vi "General Config.vi"(8 "error In":errorcluster, 10 "IOList":T2, 11 "reference":refnum<vi>) -> (0 "error out":errorcluster, 3 "Out reference":refnum<vi>)   [LabVIEW 2015]
uses:
  Control Button/Exit.ctl
  Control Button/Daq.ctl
  Control Button/Scanner config.ctl
  Control Button/Program Seq.ctl
  Control Button/cali.ctl
  Control Button/shift change.ctl
  Control Button/User mgt.ctl
  Control Button/model create.ctl
  Galobal variable_TI.vi
panel:
  in  "lvdt Setting":bool
  out "Job Id":string
  in  "image Setting":bool
  out "User Name 3":string
  in  "Model Create":T1
  in  "User Mgt":T3
  out "User Name 2":string
  in  "Shift":T4
  in  "Calibration":T5
  in  "IO List Update":bool
  out "error out 2":errorcluster
  in  "error in (no error)":errorcluster
  in  "Program Seq":T6
  in  "Scanner config":T7
  in  "DAQ Config":T8
  out "User Name":string
  in  "Exit":T9
  out "String":string
  out "appended path":path
  in  "Ring":u16(ring)
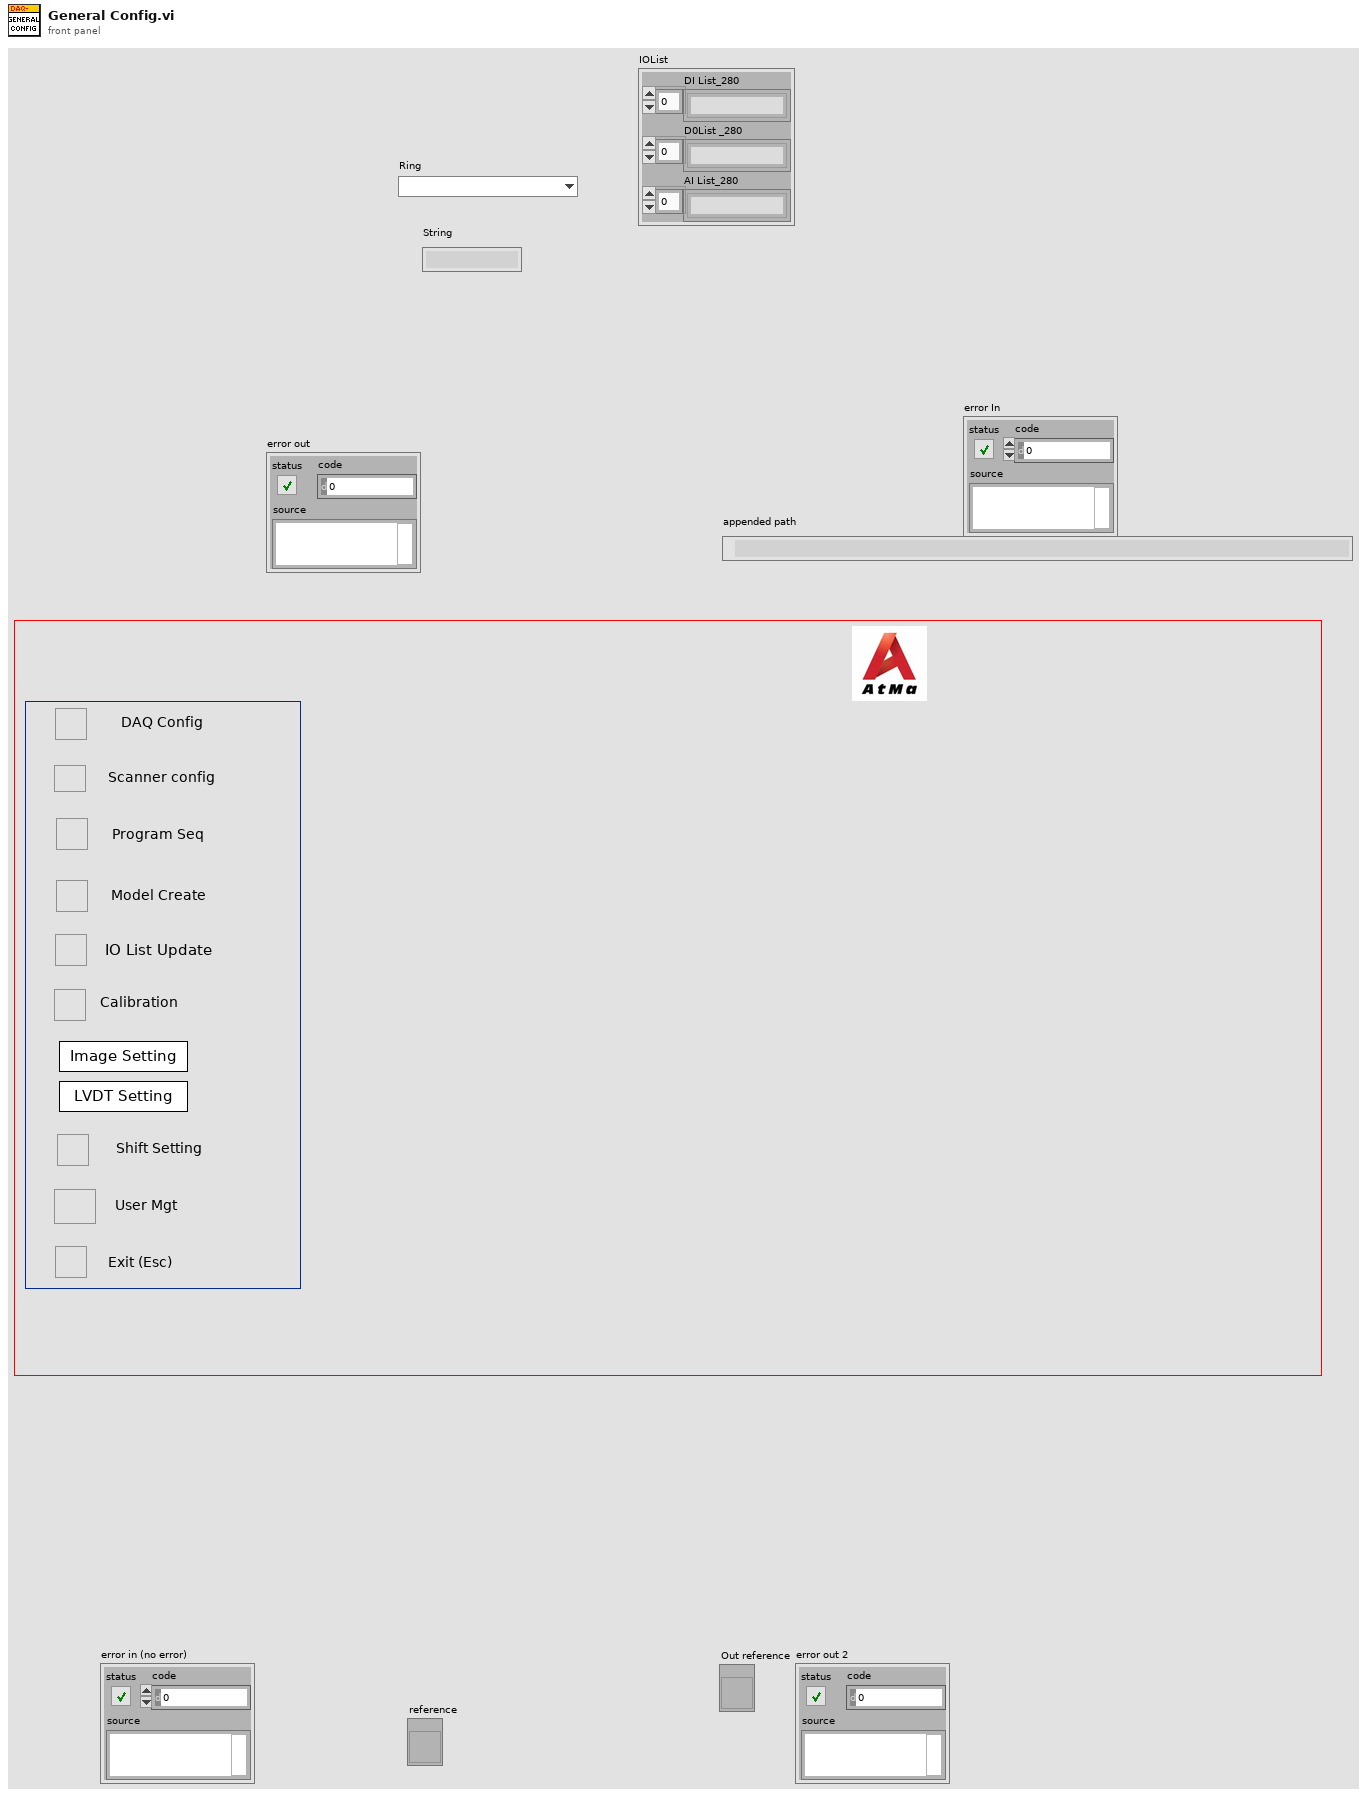
[diagram p1: front panel]
types:
  T1 = typedef "model create.ctl" = bool
  T2 = cluster{"DI List_280":string[], "D0List _280":string[], "AI List_280":string[]}
  T3 = typedef "User mgt.ctl" = bool
  T4 = typedef "shift change.ctl" = bool
  T5 = typedef "cali.ctl" = bool
  T6 = typedef "Program Seq.ctl" = bool
  T7 = typedef "Scanner config.ctl" = bool
  T8 = typedef "Daq.ctl" = bool
  T9 = typedef "Exit.ctl" = bool
  T10 = enum32{"Invalid", "Standard", "Closed", "Hidden", "Minimized", "Maximized"}
  T11 = cluster{"XInput":dbl[], "Y New Value":dbl[], "Avg point":i16}[]
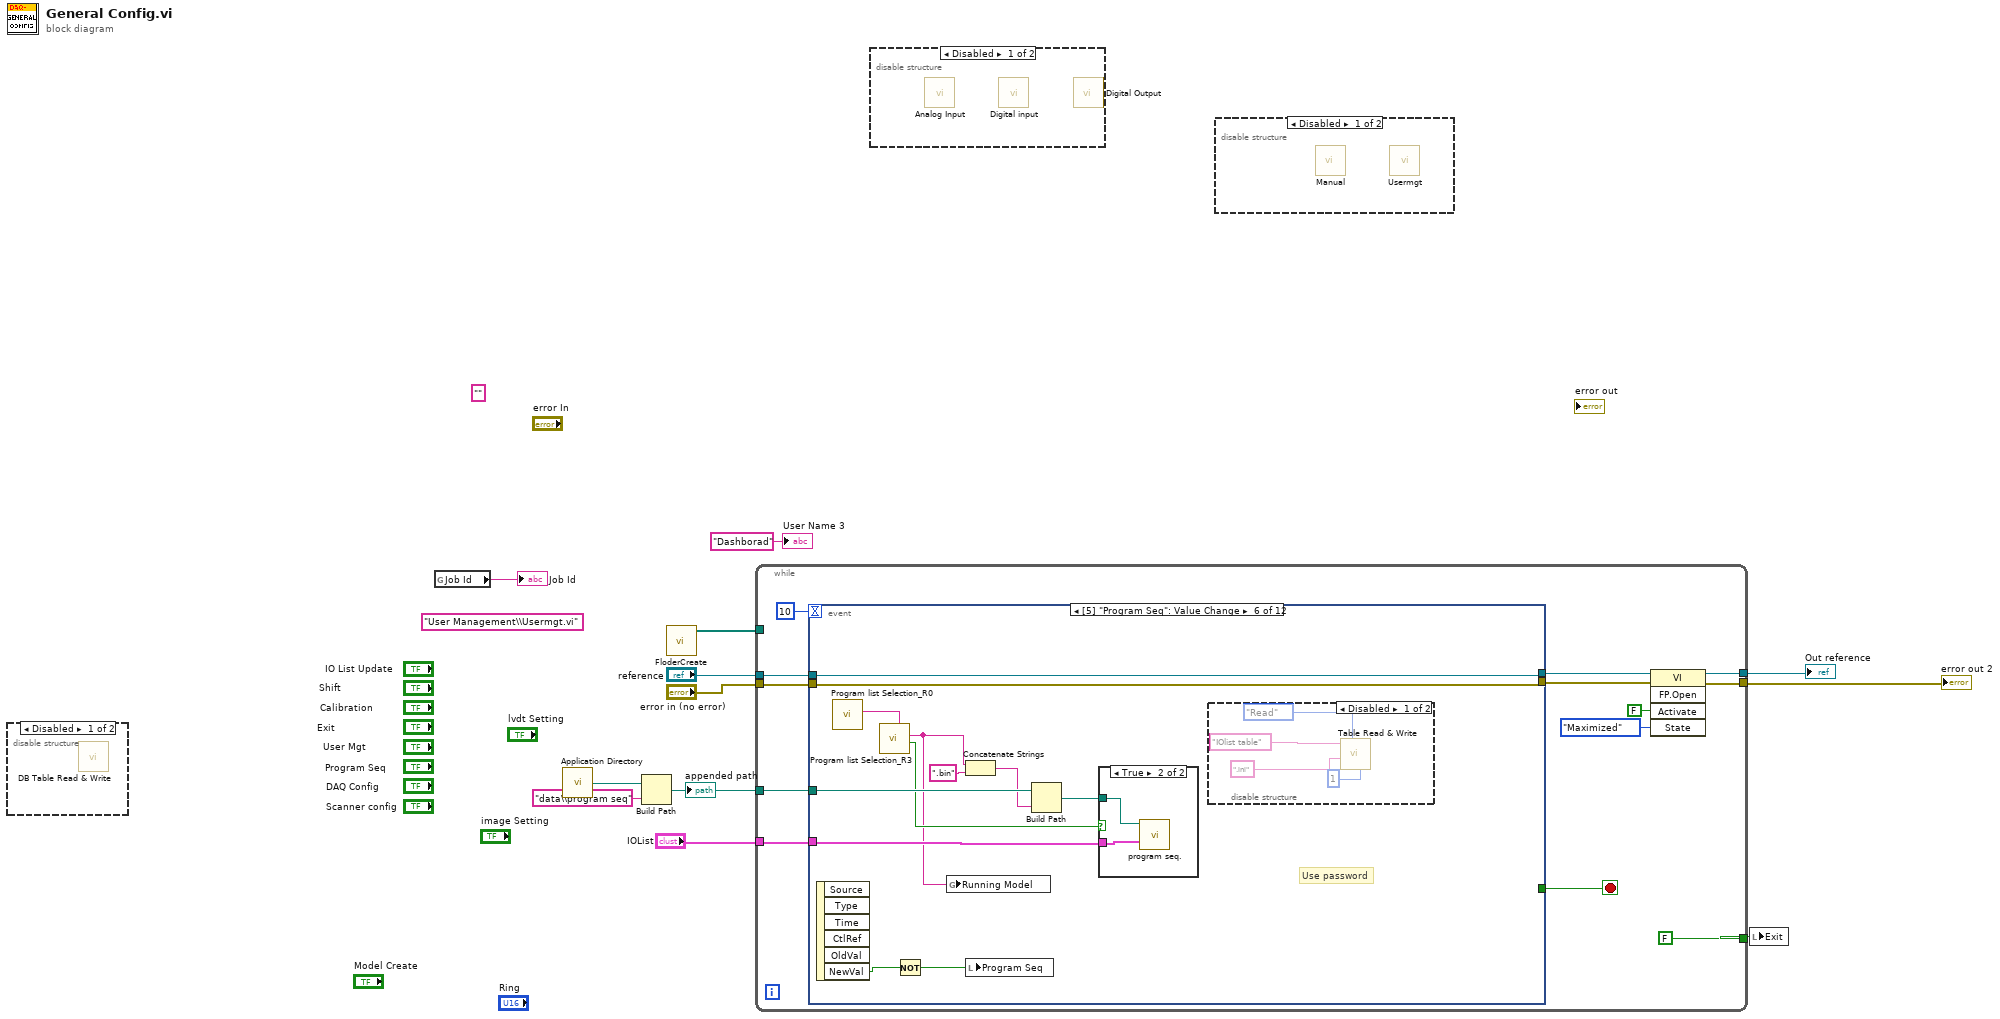
[diagram p0: block diagram]
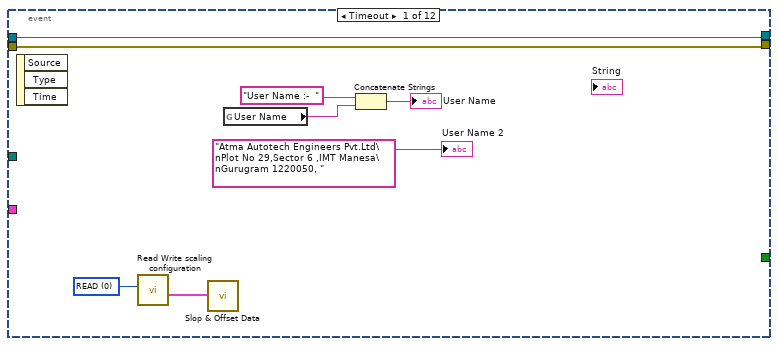
[diagram p5: hidden frame]
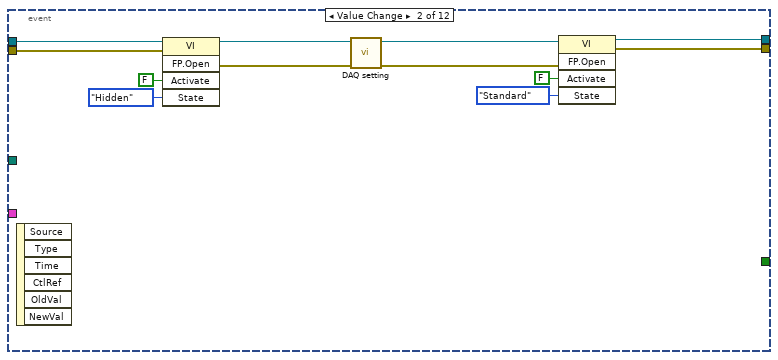
[diagram p6: hidden frame]
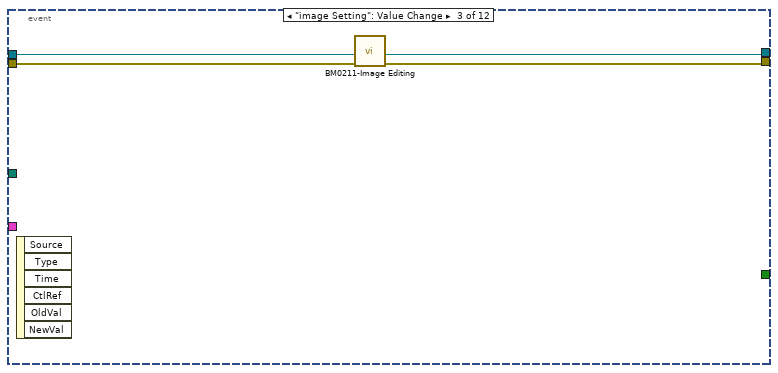
[diagram p7: hidden frame]
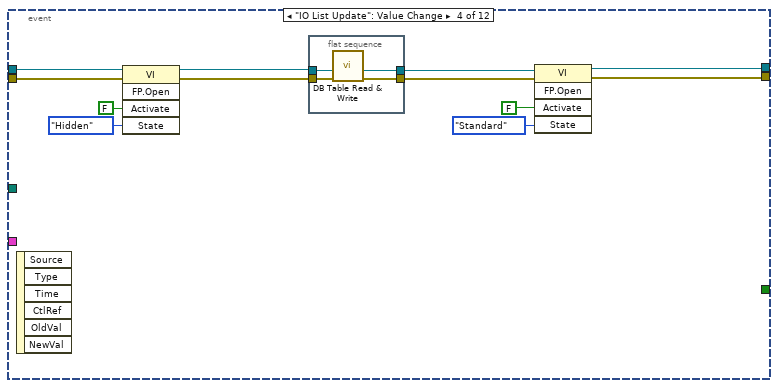
[diagram p8: hidden frame]
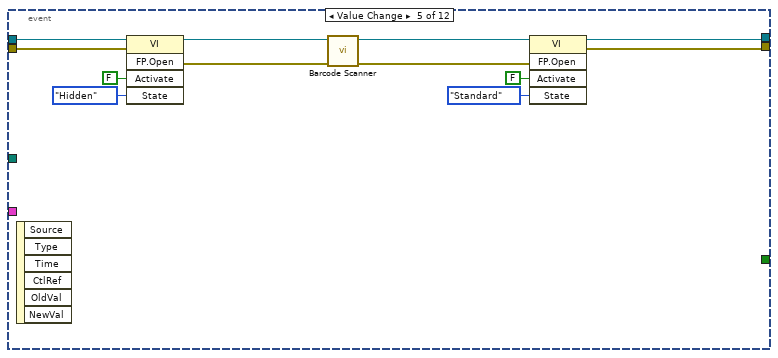
[diagram p9: hidden frame]
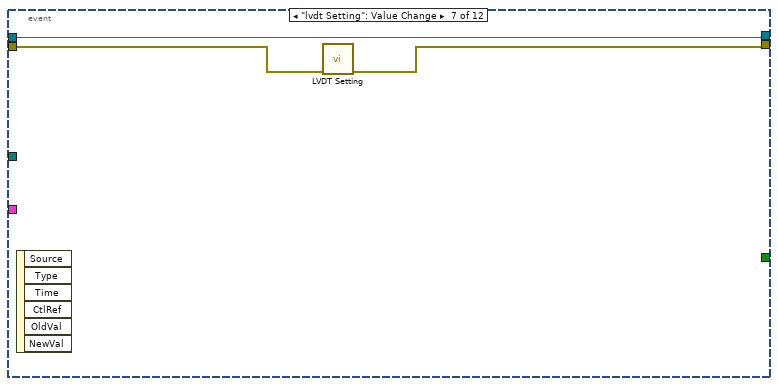
[diagram p12: hidden frame]
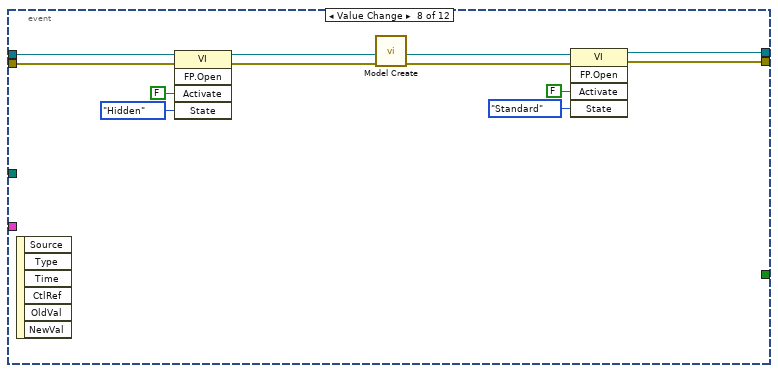
[diagram p13: hidden frame]
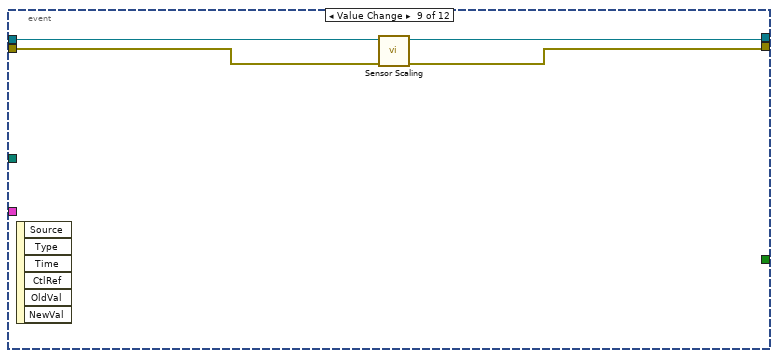
[diagram p14: hidden frame]
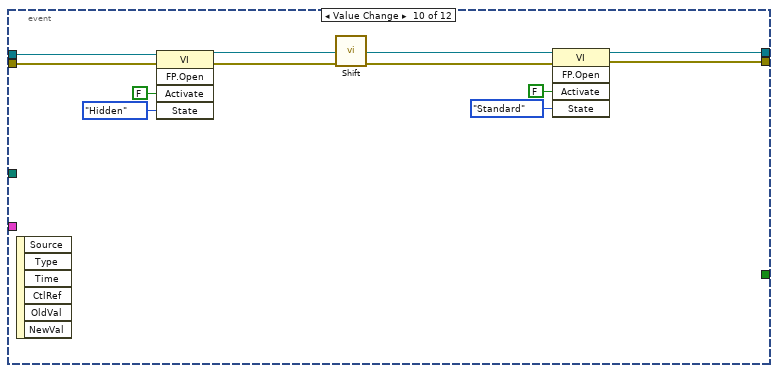
[diagram p15: hidden frame]
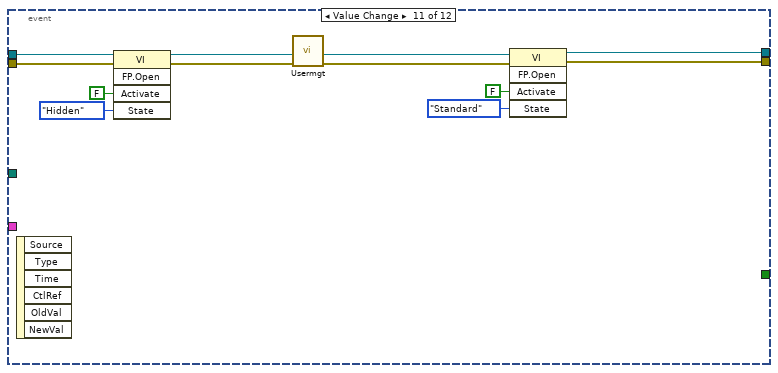
[diagram p16: hidden frame]
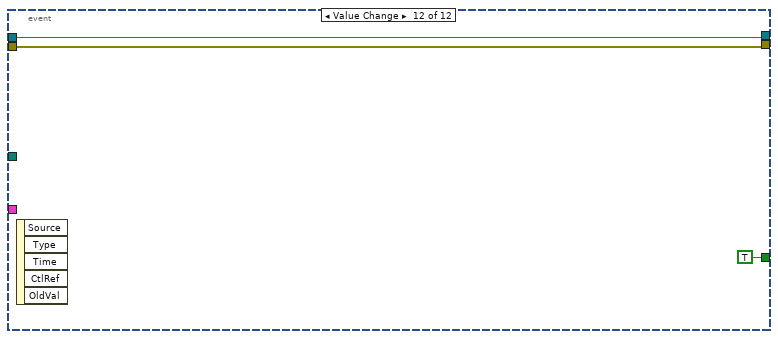
[diagram p17: hidden frame]
diagram:
  (unwired) "User Management\\Usermgt.vi" ("name or relative path")
  (unwired) ""
  n1 = disable-structure shown="Disabled" {
    frame Disabled {
      n2 = call "DB Table Read & Write.vi"() -> ()  [unwired: 10 in, 2 out]
    }
    frame Enabled {
    }
  }
  n3 = global read "Galobal variable_TI.vi" "Job Id"() -> (→"Job Id":string)
  n4 = call <vilib>:"Application Directory.vi"() -> ("Application Directory"=w6:path)
  n5 = Build Path(base path=w6, name or relative path="data\\program seq") -> (appended path=w3:path)
  "appended path" <- w3
  n6 = call "FloderCreate.vi"() -> ("File Path"=w7:path[])  [unwired: 11 in]
  n7 = while {
    tunnel: w3 -> [w13]
    tunnel: "reference" -> [w23]
    tunnel: "error in (no error)" -> [w22]
    tunnel: [w17] -> w11
    tunnel: [w16] -> w10
    tunnel: [T9 FALSE ("Exit")] -> w9
    tunnel: w7 -> [_]
    tunnel: "IOList" -> [w14]
    stop <- w24 stop-if-true
    n8 = event shown="[5] \"Program Seq\": Value Change" {
      selector: _ -> [_ _ _ _ _ _ _ _ _ _ _ _]
      dyn-events: _ -> [_ _ _ _ _ _ _ _ _ _ _ _]
      timeout: 10 -> [_ _ _ _ _ _ _ _ _ _ _ _]
      tunnel: [_ _ _ _ _ _ _ _ _ _ _ TRUE ("Exit")] -> w24
      tunnel: w23 -> [w30 w37 w48 w52 w74 w88 w97 w104 w111 w119 w128 w136]
      tunnel: w22 -> [w29 w36 w47 w51 w73 w87 w96 w103 w110 w117 w126 w135]
      tunnel: [w30 w35 w48 w59 w66 w88 w97 w99 w111 w118 w127 w136] -> w19
      tunnel: [w29 w34 w46 w58 w65 w87 w95 w98 w109 w116 w125 w135] -> w18
      tunnel: w14 -> [_ _ _ _ _ w86 _ _ _ _ _ _]
      tunnel: w13 -> [_ _ _ _ _ w85 _ _ _ _ _ _]
      event Timeout {
        w28 = u16 0 items=["READ", "WRITE"] ("Read/Write")
        n9 = event-data() -> ()  [unwired: 1 in, 3 out]
        n10 = call "Read Write scaling configuration.vi"("Read/Write"=w28) -> ("Output"=w27:T11)  [unwired: 4 in, 2 out]
        n11 = call "Slop & Offset Data.vi"("Input"=w27) -> ()  [unwired: 10 in, 1 out]
        n12 = global read "Galobal variable_TI.vi" "User Name"() -> (w33:string)
        n13 = Concatenate Strings("User Name :-  " ("string"), w33) -> (→"User Name":string)
        "User Name 2" <- "Atma Autotech Engineers Pvt.Ltd\nPlot No 29,Sector 6 ,IMT Manesa\nGurugram 1220050, " ("string")
      }
      event Value Change {
        n14 = event-data() -> ()  [unwired: 1 in, 6 out]
        n15 = invoke class="VI" method="FP.Open"(reference=w37, error in=w36, "Activate"=FALSE ("Activate?"), "State"=T10."Hidden") -> (reference out=w43:refnum<vi>, error out=w42:errorcluster)  [unwired: 1 in, 3 out]
        n16 = call "DAQ setting.vi"("error in (no error)"=w42, "vi reference"=w43) -> ("error Out"=w38:errorcluster, "Out reference"=w39:refnum<vi>)  [unwired: 8 in]
        n17 = invoke class="VI" method="FP.Open"(reference=w39, error in=w38, "Activate"=FALSE ("Activate?"), "State"=T10."Standard") -> (reference out=w35:refnum<vi>, error out=w34:errorcluster)  [unwired: 1 in, 3 out]
      }
      event "image Setting": Value Change {
        n18 = event-data() -> ()  [unwired: 1 in, 6 out]
        n19 = call "BM0211-Image Editing.vi"("error IN"=w47) -> ("error out"=w46:errorcluster)  [unwired: 10 in]
      }
      event "IO List Update": Value Change {
        n20 = event-data() -> ()  [unwired: 1 in, 6 out]
        n21 = invoke class="VI" method="FP.Open"(reference=w52, error in=w51, "Activate"=FALSE ("Activate?"), "State"=T10."Hidden") -> (reference out=w50:refnum<vi>, error out=w49:errorcluster)  [unwired: 1 in, 3 out]
        n22 = flat-sequence {
          tunnel: [w61] -> w56
          tunnel: [w62] -> w55
          tunnel: w50 -> [w63]
          tunnel: w49 -> [w64]
          frame #0 {
            n23 = call "DB Table Read & Write.vi"("error in"=w64, "reference"=w63) -> ("error out"=w61:errorcluster, "referenceOut"=w62:refnum<vi>)  [unwired: 8 in]
          }
        }
        n24 = invoke class="VI" method="FP.Open"(reference=w55, error in=w56, "Activate"=FALSE ("Activate?"), "State"=T10."Standard") -> (reference out=w59:refnum<vi>, error out=w58:errorcluster)  [unwired: 1 in, 3 out]
      }
      event Value Change {
        n25 = event-data() -> ()  [unwired: 1 in, 6 out]
        n26 = invoke class="VI" method="FP.Open"(reference=w74, error in=w73, "Activate"=FALSE ("Activate?"), "State"=T10."Hidden") -> (reference out=w70:refnum<vi>, error out=w69:errorcluster)  [unwired: 1 in, 3 out]
        n27 = call "Barcode Scanner.vi"("error in (no error)"=w69, "reference"=w70) -> ("error in (no error) 2"=w67:errorcluster, "reference 2"=w68:refnum<vi>)  [unwired: 8 in]
        n28 = invoke class="VI" method="FP.Open"(reference=w68, error in=w67, "Activate"=FALSE ("Activate?"), "State"=T10."Standard") -> (reference out=w66:refnum<vi>, error out=w65:errorcluster)  [unwired: 1 in, 3 out]
      }
      event Value Change {
        # "Use password"
        n29 = event-data() -> ("NewVal"=w81:T6)  [unwired: 1 in, 5 out]
        n30 = call "Program list Selection_R0.vi"() -> ("String"=w79:string)  [unwired: 8 in, 3 out]
        n31 = call "Program list Selection_R3.vi"("new element/subarray"=w79) -> ("Exit"=w78:bool, "String"=w77:string)  [unwired: 7 in, 2 out]
        n32 = Not(x=w81) -> (.not. x?=w80:T6)
        n33 = global write "Galobal variable_TI.vi" "Running Model"(w77) -> ()
        n34 = Concatenate Strings(w77, ".bin" ("string")) -> (w84:string)
        n35 = local write "Program Seq"(w80) -> ()
        n36 = Build Path(base path=w85, name or relative path=w84) -> (appended path=w82:path)
        n37 = case shown="True" w78 {
          tunnel: w86 -> [_ w89]
          tunnel: w82 -> [_ w90]
          frame False {
          }
          frame True {
            n38 = call "program seq..vi"("IOList"=w89, "Filepath"=w90) -> ()  [unwired: 9 in, 1 out]
          }
        }
        n39 = disable-structure shown="Disabled" {
          frame Disabled {
            n40 = call "Table Read & Write.vi"("File Name"="IOlist table", "File type"=".ini", "Enum"=enum16{"Read", "Write"}."Read", "index"=1) -> ()  [unwired: 5 in, 2 out]
          }
          frame Enabled {
          }
        }
      }
      event "lvdt Setting": Value Change {
        n41 = event-data() -> ()  [unwired: 1 in, 6 out]
        n42 = call "LVDT Setting.vi"("error in (no error)"=w96) -> ("error out 2"=w95:errorcluster)  [unwired: 10 in]
      }
      event Value Change {
        n43 = event-data() -> ()  [unwired: 1 in, 6 out]
        n44 = invoke class="VI" method="FP.Open"(reference=w104, error in=w103, "Activate"=FALSE ("Activate?"), "State"=T10."Hidden") -> (reference out=w100:refnum<vi>, error out=w102:errorcluster)  [unwired: 1 in, 3 out]
        n45 = call "Model Create.vi"("error in (no error)"=w102) -> ("error out"=w101:errorcluster)  [unwired: 10 in]
        n46 = invoke class="VI" method="FP.Open"(reference=w100, error in=w101, "Activate"=FALSE ("Activate?"), "State"=T10."Standard") -> (reference out=w99:refnum<vi>, error out=w98:errorcluster)  [unwired: 1 in, 3 out]
      }
      event Value Change {
        n47 = event-data() -> ()  [unwired: 1 in, 6 out]
        n48 = call "Sensor Scaling.vi"("error in"=w110) -> ("error out"=w109:errorcluster)  [unwired: 9 in, 1 out]
      }
      event Value Change {
        n49 = event-data() -> ()  [unwired: 1 in, 6 out]
        n50 = invoke class="VI" method="FP.Open"(reference=w119, error in=w117, "Activate"=FALSE ("Activate?"), "State"=T10."Hidden") -> (reference out=w120:refnum<vi>, error out=w122:errorcluster)  [unwired: 1 in, 3 out]
        n51 = call "Shift.vi"("error in"=w122) -> ("error out"=w121:errorcluster)  [unwired: 10 in]
        n52 = invoke class="VI" method="FP.Open"(reference=w120, error in=w121, "Activate"=FALSE ("Activate?"), "State"=T10."Standard") -> (reference out=w118:refnum<vi>, error out=w116:errorcluster)  [unwired: 1 in, 3 out]
      }
      event Value Change {
        n53 = event-data() -> ()  [unwired: 1 in, 6 out]
        n54 = invoke class="VI" method="FP.Open"(reference=w128, error in=w126, "Activate"=FALSE ("Activate?"), "State"=T10."Hidden") -> (reference out=w129:refnum<vi>, error out=w124:errorcluster)  [unwired: 1 in, 3 out]
        n55 = call "Usermgt.vi"("error In"=w124) -> ("error out"=w123:errorcluster)  [unwired: 10 in]
        n56 = invoke class="VI" method="FP.Open"(reference=w129, error in=w123, "Activate"=FALSE ("Activate?"), "State"=T10."Standard") -> (reference out=w127:refnum<vi>, error out=w125:errorcluster)  [unwired: 1 in, 3 out]
      }
      event Value Change {
        n57 = event-data() -> ()  [unwired: 1 in, 5 out]
      }
    }
    n58 = invoke class="VI" method="FP.Open"(reference=w19, error in=w18, "Activate"=FALSE ("Activate?"), "State"=T10."Maximized") -> (reference out=w17:refnum<vi>, error out=w16:errorcluster)  [unwired: 1 in, 3 out]
  }
  "Out reference" <- w11
  "error out 2" <- w10
  n59 = disable-structure shown="Disabled" {
    frame Disabled {
      n60 = call "Analog Input.vi"() -> ()  [unwired: 10 in, 2 out]
      n61 = call "Digital input.vi"() -> ()  [unwired: 10 in, 2 out]
      n62 = call "Digital Output.vi"() -> ()  [unwired: 10 in, 2 out]
    }
    frame Enabled {
    }
  }
  n63 = disable-structure shown="Disabled" {
    frame Disabled {
      n64 = call "Manual.vi"() -> ()  [unwired: 10 in, 2 out]
      n65 = call "Usermgt.vi"() -> ()  [unwired: 11 in, 1 out]
    }
    frame Enabled {
    }
  }
  n66 = local write "Exit"(w9) -> ()
  "User Name 3" <- "Dashborad" ("User Name 3")
